vi "13_Sum of first 10 Natural no.vi"() -> ()   [LabVIEW 2018]
panel:
  out "Sum=":dbl
  # "Develop a HMI to find sum of first 10 natural numbers using for loop."
  # "Shift register acts like a memory.\nMemory can be past or next."
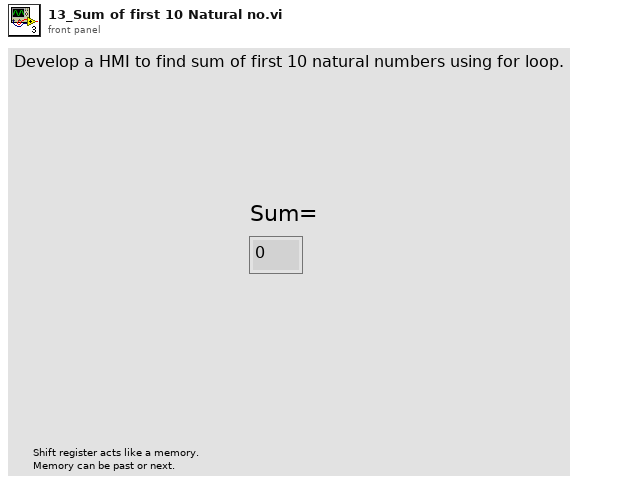
[diagram p1: front panel]
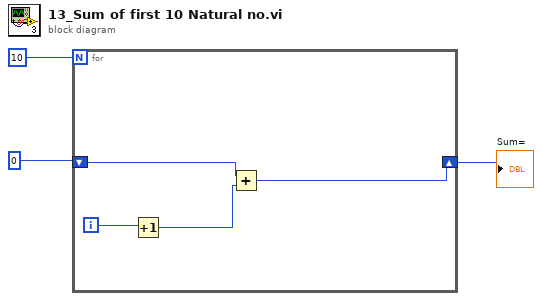
[diagram p0: block diagram]
diagram:
  n1 = for {
    N: 10 -> [_]
    shift-right: [w6] -> w1
    shift-left: 0 -> [w7]
    i -> [w5]
    n2 = Increment(x=w5) -> (x+1=w4:i32)
    n3 = Add(x=w7, y=w4) -> (x+y=w6:i32)
  }
  "Sum=" <- w1
